vi "GE 5565PIORC.DMA.Block.Clear.vi"   [LabVIEW 2020, in "GE 5565PIORC.lvclass"]
doc: "Reads <B>count</B> elements from the provided <B>Block Descriptor</B> into a newly allocated <B>data</B> array."
uses:
  GE 5565PIORC.lvclass
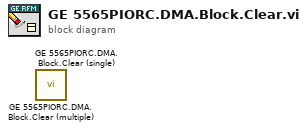
[diagram p0: block diagram]
diagram:
  n1 = call "GE 5565PIORC.DMA.Block.Clear (multiple).vi"() -> ()  [unwired: 9 in, 3 out]
  n2 = call "GE 5565PIORC.DMA.Block.Clear (single).vi"() -> ()  [unwired: 9 in, 3 out]
